vi "Packbits.vi"() -> ()   [LabVIEW 2020]
panel:
  out "Array 2":u8[](array[numeric]) format="%.0x"
  out "Array":u8[](array[numeric]) format="%.0x"
  in  "String":string
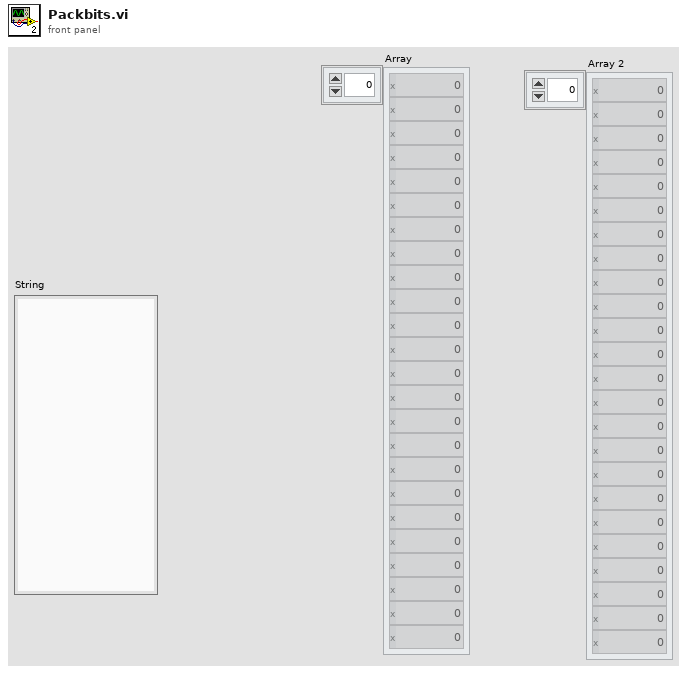
[diagram p1: front panel]
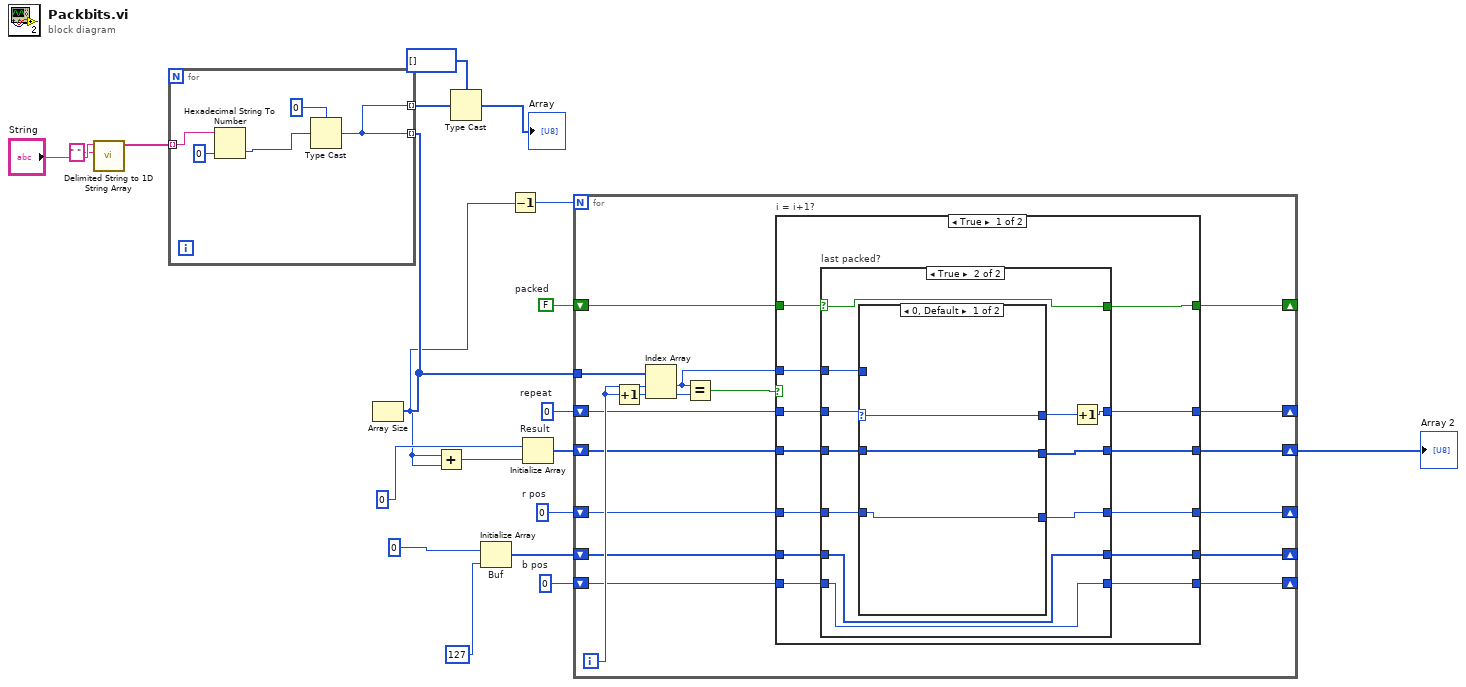
[diagram p0: block diagram]
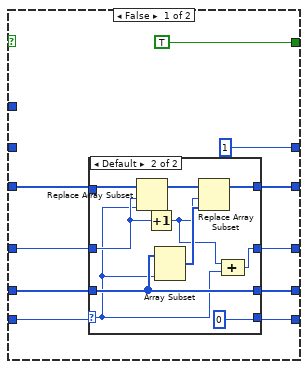
[diagram p2: hidden frame]
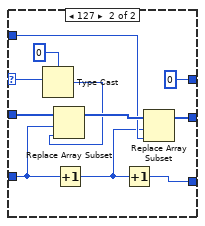
[diagram p4: hidden frame]
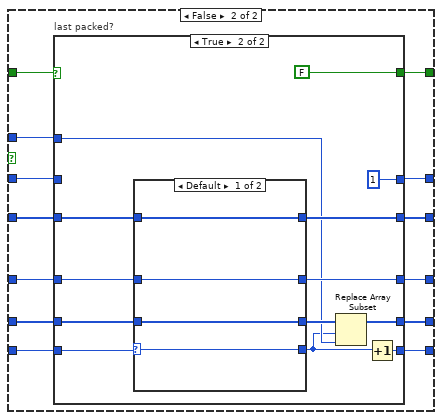
[diagram p5: hidden frame]
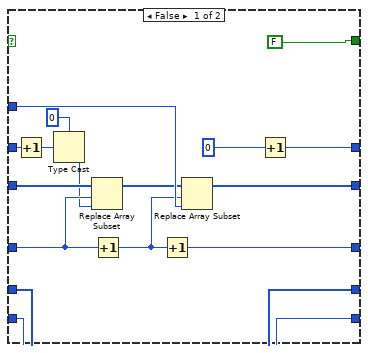
[diagram p6: hidden frame]
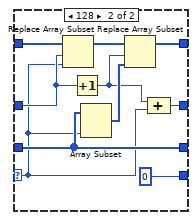
[diagram p7: hidden frame]
diagram:
  w8 = 0  # b pos
  w13 = 0  # repeat
  w14 = FALSE  # packed
  w15 = 0  # r pos
  n1 = call <vilib>:"Delimited String to 1D String Array.vi"("delimiter"=" ", "delimited string"="String") -> ("string array"=w18:string[])  [unwired: 9 in]
  n2 = for {
    tunnel: w18 -> [w25] mode=indexing
    tunnel: [w22] -> w17 mode=indexing
    tunnel: [w22] -> w4 mode=indexing
    n3 = Hexadecimal String To Number(string=w25, default (0uL)=u8 0 ("default (0 U32)")) -> (number=w23:u8)  [unwired: 1 in, 1 out]
    n4 = Type Cast(type=i8 0, x=w23) -> (*(type *) &x=w22:i8)
  }
  n5 = Array Size(array=w17) -> (size(s)=w6:i32)
  n6 = Add(x=w6, y=w6) -> (x+y=w7:i32)
  n7 = Type Cast(type=u8[] [], x=w4) -> (*(type *) &x=→"Array":u8[])
  n8 = Initialize Array "Buf"(i8 0, 127 ("dimension size")) -> (w9:i8[])
  n9 = Decrement(x=w6) -> (x-1=w12:i32)
  n10 = Initialize Array "Result"(i8 0, w7) -> (w16:i8[])
  n11 = for {
    N: w12 -> [_]
    tunnel: w17 -> [w43]
    shift-right: [w30] -> w3
    shift-left: w16 -> [w29]
    shift-right: [w28] -> _
    shift-left: w15 -> [w27]
    shift-right: [w38] -> _
    shift-left: w14 -> [w37]
    shift-right: [w34] -> _
    shift-left: w13 -> [w33]
    shift-right: [w36] -> _
    shift-left: w9 -> [w35]
    shift-right: [w32] -> _
    shift-left: w8 -> [w31]
    i -> [w42]
    n12 = Increment(x=w42) -> (x+1=w41:i32)
    n13 = Index Array(array=w43, index #1=w42, index #2=w41) -> (element #1=w26:i8, element #2=w40:i8)
    n14 = Equal?(x=w26, y=w40) -> (x = y?=w39:bool)
    n15 = case "i = i+1?" shown="True" w39 {
      tunnel: [w55 w117] -> w38
      tunnel: w37 -> [w56 w118]
      tunnel: [w54 w116] -> w36
      tunnel: w35 -> [w53 w115]
      tunnel: [w52 w114] -> w34
      tunnel: w33 -> [w51 w113]
      tunnel: [w50 w112] -> w32
      tunnel: w31 -> [w49 w111]
      tunnel: [w48 w110] -> w30
      tunnel: w29 -> [w47 w109]
      tunnel: [w46 w108] -> w28
      tunnel: w27 -> [w45 w107]
      tunnel: w26 -> [w44 w106]
      frame True {
        n16 = case "last packed?" shown="True" w56 {
          selector: w56 -> [_ w81]
          tunnel: [TRUE w81] -> w55
          tunnel: [w57 w83] -> w54
          tunnel: w53 -> [w62 w83]
          tunnel: [1 ("repeat") w85] -> w52
          tunnel: w51 -> [_ w91]
          tunnel: [w60 w82] -> w50
          tunnel: w49 -> [w61 w82]
          tunnel: [w63 w89] -> w48
          tunnel: w47 -> [w64 w88]
          tunnel: [w59 w87] -> w46
          tunnel: w45 -> [w58 w86]
          tunnel: w44 -> [_ w84]
          frame False {
            n17 = case shown="Default" w61 {
              selector: w61 -> [w67 w71]
              tunnel: w64 -> [w70 w80]
              tunnel: [w70 w78] -> w63
              tunnel: w58 -> [w69 w75]
              tunnel: w62 -> [w68 w74]
              tunnel: [w67 0 ("b pos")] -> w60
              tunnel: [w69 w73] -> w59
              tunnel: [w68 w74] -> w57
              frame 0 {
              }
              frame Default {
                n18 = Replace Array Subset(array=w80, new element=w71, index=w75) -> (w79:i8[])
                n19 = Increment(x=w75) -> (x+1=w72:i32)
                n20 = Array Subset(array=w74, length=w71) -> (w77:i8[])  [unwired: 1 in]
                n21 = Replace Array Subset(array=w79, new element=w77, index=w72) -> (w78:i8[])
                n22 = Compound Arithmetic op=ADD(w72, w71) -> (w73:i32)
              }
            }
          }
          frame True {
            n23 = case shown="0, Default" w91 {
              selector: w91 -> [w94 w102]
              tunnel: [w94 0 ("repeat")] -> w90
              tunnel: [w93 w99] -> w89
              tunnel: w88 -> [w93 w104]
              tunnel: [w92 w95] -> w87
              tunnel: w86 -> [w92 w97]
              tunnel: w84 -> [_ w98]
              frame 0, Default {
              }
              frame 127 {
                n24 = Type Cast(type=i8 0, x=w102) -> (*(type *) &x=w100:i8)
                n25 = Replace Array Subset(array=w104, new element=w100, index=w97) -> (w101:i8[])
                n26 = Increment(x=w97) -> (x+1=w96:i32)
                n27 = Increment(x=w96) -> (x+1=w95:i32)
                n28 = Replace Array Subset(array=w101, new element=w98, index=w96) -> (w99:i8[])
              }
            }
            n29 = Increment(x=w90) -> (x+1=w85:i32)
          }
        }
      }
      frame False {
        n30 = case "last packed?" shown="True" w118 {
          tunnel: [FALSE FALSE] -> w117
          tunnel: [w126 w138] -> w116
          tunnel: w115 -> [w126 w143]
          tunnel: [w128 1 ("repeat")] -> w114
          tunnel: w113 -> [w134 _]
          tunnel: [w125 w135] -> w112
          tunnel: w111 -> [w125 w142]
          tunnel: [w132 w144] -> w110
          tunnel: w109 -> [w131 w145]
          tunnel: [w130 w141] -> w108
          tunnel: w107 -> [w129 w140]
          tunnel: w106 -> [w127 w137]
          frame False {
            n31 = Increment(x=w134) -> (x+1=w120:i32)
            n32 = Type Cast(type=i8 0, x=w120) -> (*(type *) &x=w122:i8)
            n33 = Replace Array Subset(array=w131, new element=w122, index=w129) -> (w123:i8[])
            n34 = Increment(x=w129) -> (x+1=w121:i32)
            n35 = Increment(x=w121) -> (x+1=w130:i32)
            n36 = Replace Array Subset(array=w123, new element=w127, index=w121) -> (w132:i8[])
            n37 = Increment(x=0 ("repeat")) -> (x+1=w128:i32)
          }
          frame True {
            n38 = case shown="Default" w142 {
              selector: w142 -> [w148 w152]
              tunnel: w145 -> [w151 w161]
              tunnel: [w151 w159] -> w144
              tunnel: w140 -> [w150 w156]
              tunnel: w143 -> [w149 w155]
              tunnel: [w148 0 ("b pos")] -> w136
              tunnel: [w150 w154] -> w141
              tunnel: [w149 w155] -> w139
              frame Default {
              }
              frame 128 {
                n39 = Replace Array Subset(array=w161, new element=w152, index=w156) -> (w160:i8[])
                n40 = Increment(x=w156) -> (x+1=w153:i32)
                n41 = Array Subset(array=w155, length=w152) -> (w158:i8[])  [unwired: 1 in]
                n42 = Replace Array Subset(array=w160, new element=w158, index=w153) -> (w159:i8[])
                n43 = Compound Arithmetic op=ADD(w153, w152) -> (w154:i32)
              }
            }
            n44 = Replace Array Subset(array=w139, new element=w137, index=w136) -> (w138:i8[])
            n45 = Increment(x=w136) -> (x+1=w135:i32)
          }
        }
      }
    }
  }
  "Array 2" <- w3
